vi "Sub01_1_BorderFinder.vi"(10 "Border":T1, 11 "image data":T2) -> (1 "Numeric 3":i32, 2 "Numeric 2":u32, 3 "Numeric 4":i32, 4 "Numeric":u32)   [LabVIEW 2019]
uses:
  <vilib>/picture/picture.llb/imagedata.ctl
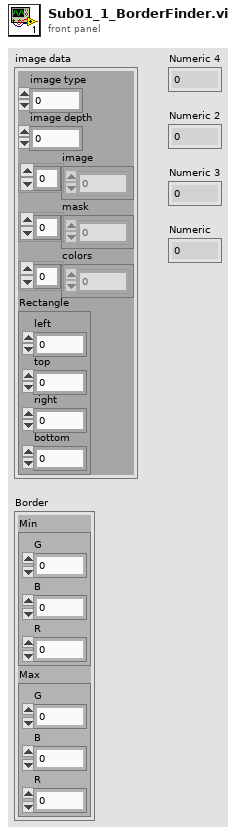
[diagram p1: front panel]
types:
  T1 = cluster{"Min":cluster{"G":u32, "B":u32, "R":u32}, "Max":cluster{"G":u32, "B":u32, "R":u32}}
  T2 = typedef "imagedata.ctl" = cluster{"image type":i32, "image depth":i32, "image":u8[], "mask":u8[], "colors":u32[], "Rectangle":cluster{"left":i16, "top":i16, "right":i16, "bottom":i16}}
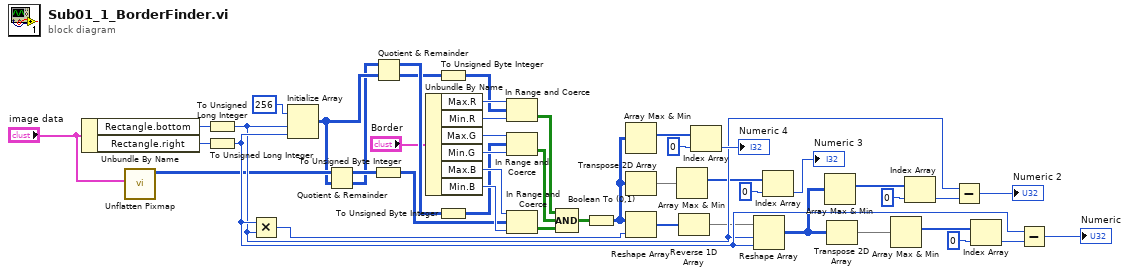
[diagram p0: block diagram]
diagram:
  n1 = Unbundle By Name("image data") -> ("Rectangle.bottom"=w24:i16, "Rectangle.right"=w41:i16)
  n2 = call <vilib>:"Unflatten Pixmap.vi"("image data"="image data") -> ("24-bit pixmap"=w11:u32[][])  [unwired: 4 in, 6 out]
  n3 = To Unsigned Long Integer(number=w24) -> (unsigned 32bit integer=w33:u32)
  n4 = To Unsigned Long Integer(number=w41) -> (unsigned 32bit integer=w40:u32)
  n5 = Multiply(x=w40, y=w33) -> (x*y=w17:u32)
  n6 = Initialize Array(u32 256 ("element"), w33, w40) -> (w7:u32[][])
  n7 = Quotient & Remainder(x=w11, y=w7) -> (x-y*floor(x/y)=w6:u32[][], floor(x/y)=w3:u32[][])
  n8 = To Unsigned Byte Integer(number=w6) -> (unsigned 8bit integer=w8:u8[][])
  n9 = Quotient & Remainder(x=w3, y=w7) -> (x-y*floor(x/y)=w5:u32[][], floor(x/y)=w4:u32[][])
  n10 = Unbundle By Name("Border") -> ("Max.R"=w42:u32, "Min.R"=w43:u32, "Max.G"=w44:u32, "Min.G"=w45:u32, "Max.B"=w46:u32, "Min.B"=w47:u32)
  n11 = To Unsigned Byte Integer(number=w4) -> (unsigned 8bit integer=w10:u8[][])
  n12 = To Unsigned Byte Integer(number=w5) -> (unsigned 8bit integer=w9:u8[][])
  n13 = In Range and Coerce(upper limit=w42, x=w10, lower limit=w43) -> (In Range?=w13:bool[][])  [unwired: 1 out]
  n14 = In Range and Coerce(upper limit=w44, x=w9, lower limit=w45) -> (In Range?=w14:bool[][])  [unwired: 1 out]
  n15 = In Range and Coerce(upper limit=w46, x=w8, lower limit=w47) -> (In Range?=w15:bool[][])  [unwired: 1 out]
  n16 = Compound Arithmetic op=AND(w13, w14, w15) -> (w16:bool[][])
  n17 = Boolean To (0,1)(Boolean=w16) -> (0, 1=w22:i16[][])
  n18 = Array Max & Min(array=w22) -> (max index (indices)=w29:i32[])  [unwired: 3 out]
  n19 = Transpose 2D Array(2D array=w22) -> (transposed array=w19:i16[][])
  n20 = Reshape Array(w22, w17) -> (w21:i16[])
  n21 = Array Max & Min(array=w19) -> (max index (indices)=w30:i32[])  [unwired: 3 out]
  n22 = Reverse 1D Array(array=w21) -> (reversed array=w18:i16[])
  n23 = Index Array(array=w29, index=0) -> (element=→"Numeric 4":i32)
  n24 = Reshape Array(w18, w33, w40) -> (w23:i16[][])
  n25 = Index Array(array=w30, index=0) -> (element=→"Numeric 3":i32)
  n26 = Array Max & Min(array=w23) -> (max index (indices)=w32:i32[])  [unwired: 3 out]
  n27 = Transpose 2D Array(2D array=w23) -> (transposed array=w20:i16[][])
  n28 = Array Max & Min(array=w20) -> (max index (indices)=w31:i32[])  [unwired: 3 out]
  n29 = Index Array(array=w32, index=0) -> (element=w36:i32)
  n30 = Subtract(x=w33, y=w36) -> (x-y=→"Numeric 2":u32)
  n31 = Index Array(array=w31, index=0) -> (element=w38:i32)
  n32 = Subtract(x=w40, y=w38) -> (x-y=→"Numeric":u32)
